vi "main.vi"() -> ()   [LabVIEW 2020]
uses:
  <vilib>/sklein/WebView2/Webview2 Control/WebView2 Control.xctl
  <vilib>/sklein/WebView2/Webview2 Control/Core Env Options.ctl
  <vilib>/sklein/WebView2/Webview2 Control/Paths.ctl
  <vilib>/MediaMongrels Ltd/WebSockets/Sockets/VISA TCP Listener/VISA TCP Listener.lvclass
  <vilib>/MediaMongrels Ltd/WebSockets/WebSockets/WebSocket Server/WebSocket Server.lvclass
  <vilib>/Thomas Zilliox/LabVIEW UI Testing/ui-testing.lvlib
panel:
  out "number":dbl
  in  "WebView2 Control":string(xcontrol)
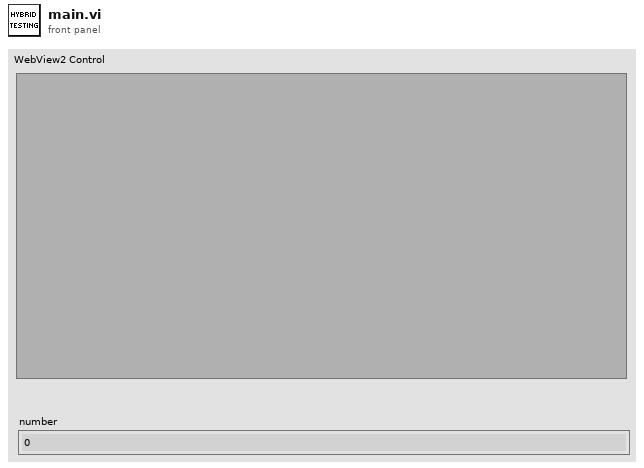
[diagram p1: front panel]
types:
  T1 = typedef "WebView2 Control.xctl/Core Env Options.ctl" = cluster{"additionalBrowserArguments":string, "language":string, "targetCompatibleBrowserVersion":string, "allowSingleSignOnUsingOSPrimaryAccount":bool}
  T2 = typedef "WebView2 Control.xctl/Paths.ctl" = cluster{"Webview2 Native":path, "Edge Application":path, "User Data":path}
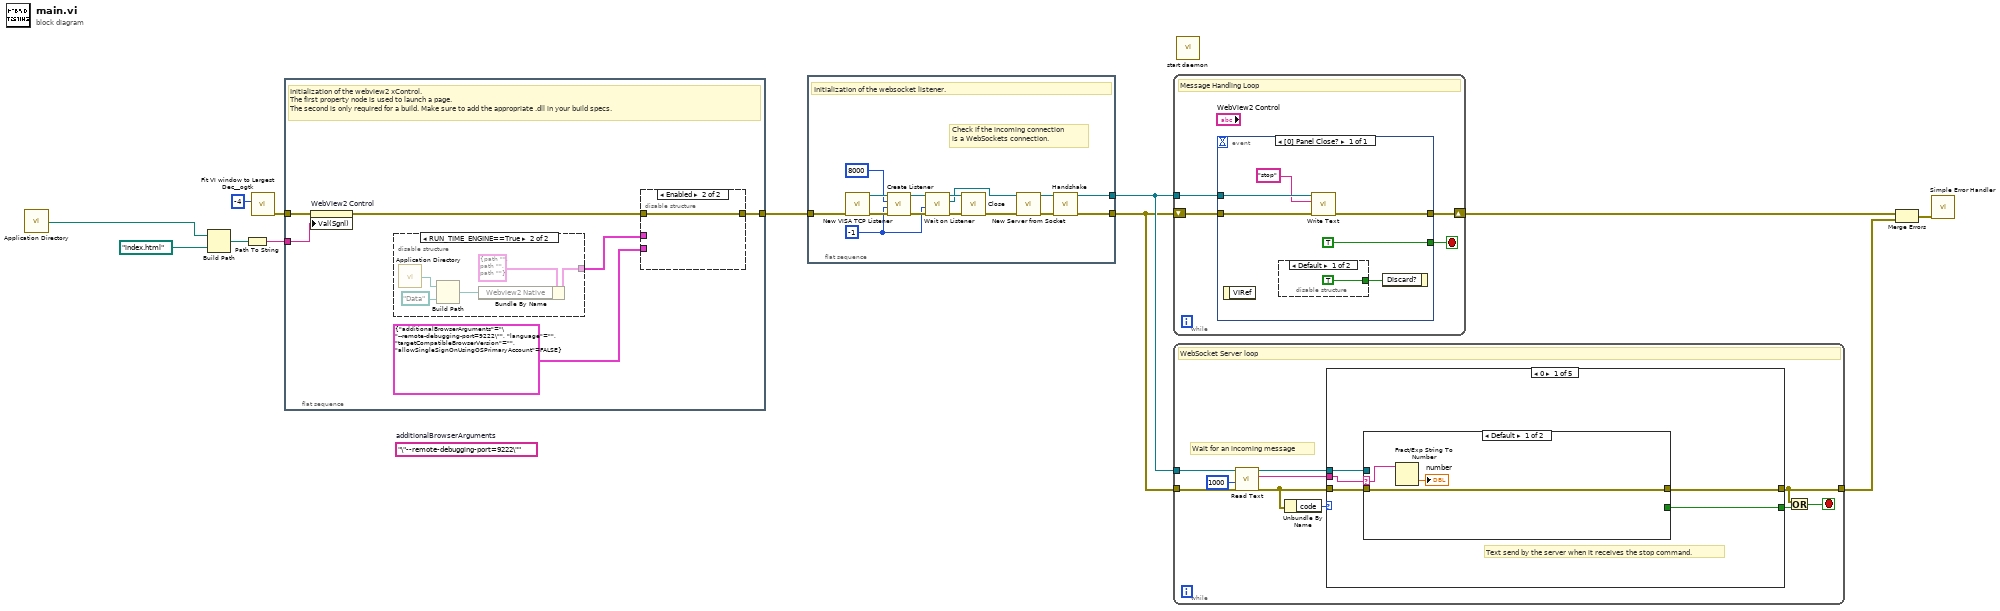
[diagram p0: block diagram]
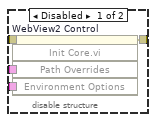
[diagram p2: hidden frame]
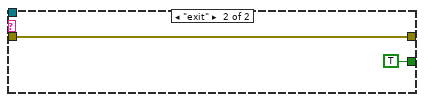
[diagram p4: hidden frame]
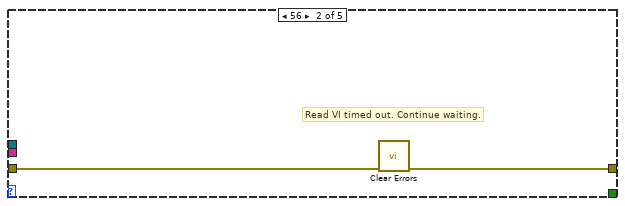
[diagram p5: hidden frame]
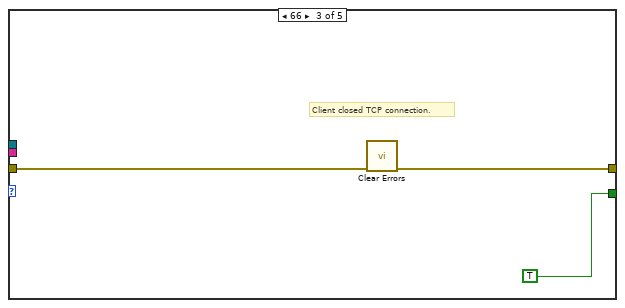
[diagram p6: hidden frame]
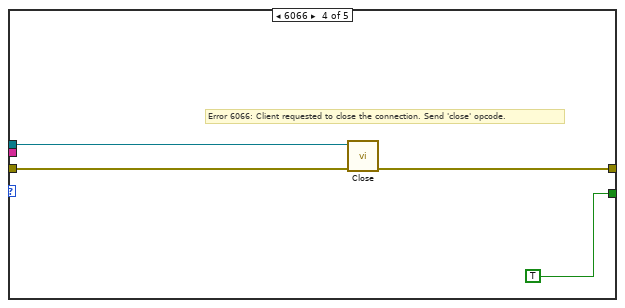
[diagram p7: hidden frame]
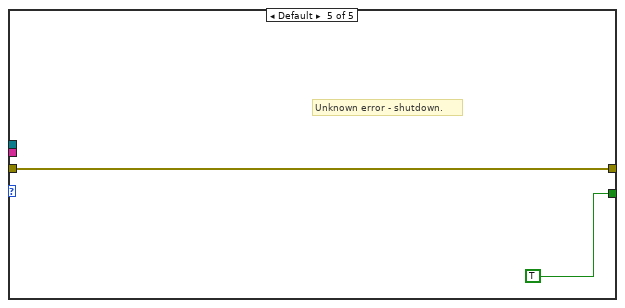
[diagram p8: hidden frame]
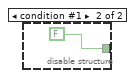
[diagram p9: hidden frame]
diagram:
  (unwired) "\"--remote-debugging-port=9222\""  # additionalBrowserArguments
  n1 = call <vilib>:"Application Directory.vi"() -> ("Application Directory"=w12:path)
  n2 = Build Path(base path=w12, name or relative path=path "index.html") -> (appended path=w11:path)
  n3 = Path To String(path=w11) -> (string=w7:string)
  n4 = call <userlib>:"Fit VI window to Largest Dec__ogtk.vi"("border spacing (2 px)"=-4) -> ("error out"=w3:errorcluster)  [unwired: 5 in, 1 out]
  n5 = flat-sequence {
    tunnel: w7 -> [w18]
    tunnel: [w16] -> w4
    tunnel: w3 -> [w14]
    frame #0 {
      # "Initialization of the webview2 xControl.\nThe first property node is used to launch a page.\nThe second is only required for a build. Make sure to add the appropriate .dll in your build specs."
      n6 = property on="WebView2 Control" class="WebView2 Control (strict)"(error in=w14, "Val(Sgnl)"=w18) -> (error out=w17:errorcluster)  [unwired: 1 in, 1 out]
      n7 = disable-structure shown="RUN_TIME_ENGINE==True" {
        disable-tunnel: [_ w27] -> w15
        frame condition #0 (active) {
        }
        frame condition #1 {
          n8 = call <vilib>:"Application Directory.vi"() -> ("Application Directory"=w26:path)
          n9 = Build Path(base path=w26, name or relative path=path "Data") -> (appended path=w24:path)
          n10 = Bundle By Name(cluster=T2 {"Webview2 Native"=path "", "Edge Application"=path "", "User Data"=path ""} ("Path Overrides"), "Webview2 Native"=w24) -> (w27:T2)
        }
      }
      n11 = disable-structure shown="Enabled" {
        disable-tunnel: w17 -> [w22 w23]
        disable-tunnel: [w21 w23] -> w16
        disable-tunnel: w15 -> [w20 _]
        disable-tunnel: T1 {"additionalBrowserArguments"="\"--remote-debugging-port=9222\"", "language"="", "targetCompatibleBrowserVersion"="", "allowSingleSignOnUsingOSPrimaryAccount"=FALSE} ("Environment Options") -> [w19 _]
        frame Disabled {
          n12 = invoke on="WebView2 Control" class="WebView2 Control (strict)" method="Init Core.vi"(error in=w22, "Path Overrides"=w20, "Environment Options"=w19) -> (error out=w21:errorcluster)  [unwired: 2 in, 4 out]
        }
        frame Enabled {
        }
      }
    }
  }
  n13 = flat-sequence {
    tunnel: [w31] -> w1
    tunnel: [w30] -> w6
    tunnel: w4 -> [w29]
    frame #0 {
      w34 = -1 ("timeout ms (25000)")
      # "Check if the incoming connection\nis a WebSockets connection."
      # "Initialization of the websocket listener."
      n14 = call <vilib>:"New VISA TCP Listener.vi"("error in (no error)"=w29) -> ("error out"=w40:errorcluster, "VISA TCP Listener out"=w41:refnum<class "VISA TCP Listener.lvclass">)  [unwired: 9 in]
      n15 = call-dynamic "Create Listener.vi"("error in (no error)"=w40, "timeout ms (5000)"=w34, "Port"=u16 8000 ("port"), "VISA TCP Listener in"=w41) -> ("error out"=w38:errorcluster, "VISA TCP Listener out"=w36:refnum<class "VISA TCP Listener.lvclass">)  [unwired: 6 in]
      n16 = call-dynamic "Wait on Listener.vi"("error in (no error)"=w38, "timeout ms (5000)"=w34, "VISA TCP Listener in"=w36) -> ("error out"=w39:errorcluster, "Socket out"=w33:refnum<class "Socket.lvclass">, "VISA TCP Listener out"=w37:refnum<class "VISA TCP Listener.lvclass">)  [unwired: 6 in]
      n17 = call-dynamic "Close.vi"("error in (no error)"=w39, "VISA TCP Listener in"=w37) -> ("error out"=w32:errorcluster)  [unwired: 9 in]
      n18 = call <vilib>:"New Server from Socket.vi"("error in (no error)"=w32, "Socket"=w33) -> ("error out"=w42:errorcluster, "WebSocket Server out"=w43:refnum<class "WebSocket Server.lvclass">)  [unwired: 8 in]
      n19 = call-dynamic "Handshake.vi"("error in (no error)"=w42, "WebSocket Connection in"=w43) -> ("error out"=w31:errorcluster, "WebSocket Connection out"=w30:refnum<class "WebSocket Server.lvclass">)  [unwired: 8 in]
    }
  }
  n20 = while {
    shift-right: [w45] -> w9
    shift-left: w1 -> [w46]
    tunnel: w6 -> [w44]
    stop <- w47 stop-if-true
    # "Message Handling Loop"
    n21 = event shown="[0] Panel Close?" {
      selector: _ -> [_]
      dyn-events: _ -> [_]
      timeout: _ -> [_]
      tunnel: [TRUE] -> w47
      tunnel: w46 -> [w50]
      tunnel: [w49] -> w45
      tunnel: w44 -> [w51]
      event Panel Close? {
        n22 = event-data() -> ()  [unwired: 1 in, 1 out]
        n23 = disable-structure shown="Default" {
          disable-tunnel: [TRUE FALSE] -> w53
          frame condition #0 (active) {
          }
          frame condition #1 {
          }
        }
        n24 = call-dynamic "Write Text.vi"("error in (no error)"=w50, "String Data"="stop", "WebSocket in"=w51) -> ("error out"=w49:errorcluster)  [unwired: 7 in, 1 out]
        n25 = event-data("Discard?"=w53) -> ()  [unwired: 1 in, 1 out]
      }
    }
  }
  n26 = while "Read Loop" {
    tunnel: w6 -> [w65]
    tunnel: [w58] -> w10
    tunnel: w1 -> [w59]
    stop <- w56 stop-if-true
    # "Wait for an incoming message"
    # "WebSocket Server loop"
    n27 = call-dynamic "Read Text.vi"("error in (no error)"=w59, "timeout ms (5000)"=1000 ("timeout ms (25000)"), "WebSocket in"=w65) -> ("error out"=w60:errorcluster, "Data"=w62:string, "WebSocket out"=w61:refnum<class "WebSocket Server.lvclass">)  [unwired: 6 in]
    n28 = Unbundle By Name(w60) -> ("code"=w63:i32)
    n29 = case shown="0" w63 {
      tunnel: w62 -> [w66 _ _ _ _]
      tunnel: [w69 _ TRUE TRUE TRUE] -> w57
      tunnel: w61 -> [w70 _ _ w84 _]
      tunnel: w60 -> [w68 w77 w79 w82 w85]
      tunnel: [w67 w76 w78 w81 w85] -> w58
      frame 0 {
        # "Text send by the server when it receives the stop command."
        n30 = case shown="Default" w66 {
          selector: w66 -> [w72 _]
          tunnel: w70 -> [_ _]
          tunnel: [_ TRUE] -> w69
          tunnel: w68 -> [w73 w75]
          tunnel: [w73 w75] -> w67
          frame Default {
            n31 = Fract/Exp String To Number(string=w72) -> (number=→"number":dbl)  [unwired: 3 in, 1 out]
          }
          frame "exit" {
          }
        }
      }
      frame 56 {
        # "Read VI timed out. Continue waiting."
        n32 = call <vilib>:"Clear Errors.vi"("error in (no error)"=w77) -> ("error out"=w76:errorcluster)  [unwired: 5 in, 1 out]
      }
      frame 66 {
        # "Client closed TCP connection."
        n33 = call <vilib>:"Clear Errors.vi"("error in (no error)"=w79) -> ("error out"=w78:errorcluster)  [unwired: 5 in, 1 out]
      }
      frame 6066 {
        # "Error 6066: Client requested to close the connection. Send 'close' opcode."
        n34 = call-dynamic "Close.vi"("error in (no error)"=w82, "WebSocket in"=w84) -> ("error out"=w81:errorcluster)  [unwired: 9 in]
      }
      frame Default {
        # "Unknown error - shutdown."
      }
    }
    n35 = Or(x=w58, y=w57) -> (x .or. y?=w56:bool)
  }
  n36 = call <vilib>:"start daemon.vi"() -> ()  [unwired: 11 in, 1 out]
  n37 = Merge Errors(w9, w10) -> (w5:errorcluster)
  n38 = call <vilib>:"Simple Error Handler.vi"("error in (no error)"=w5) -> ()  [unwired: 4 in, 5 out]
